vi "OP600ZP_CLUSTER_SOFTS_FIN.vi"(10 "MESURES":T1, 11 "EmptyTab":string[][](array[string])) -> (4 "Tab1":string[][](array[string]), 6 "PASS/FAIL":bool[](array[boolean]))   [LabVIEW 2020]
uses:
  VG/IS30%.vi
  OP600ZP_VGConf.vi
panel:
  out "VG IS30% ?":bool
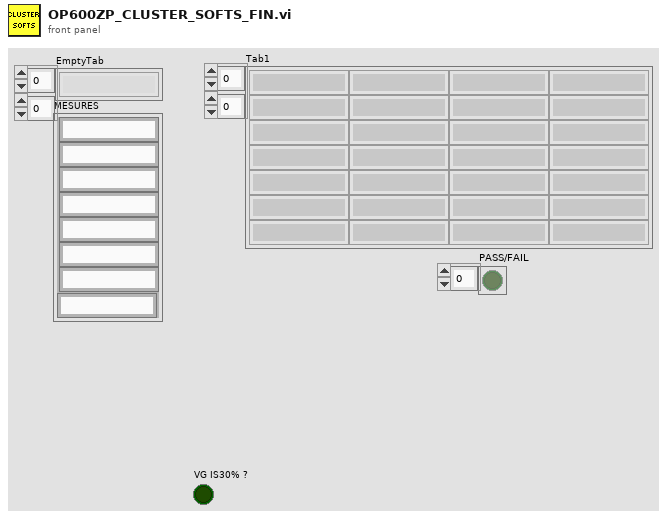
[diagram p1: front panel]
types:
  T1 = cluster{string, string, string, string, string, string, string, string}
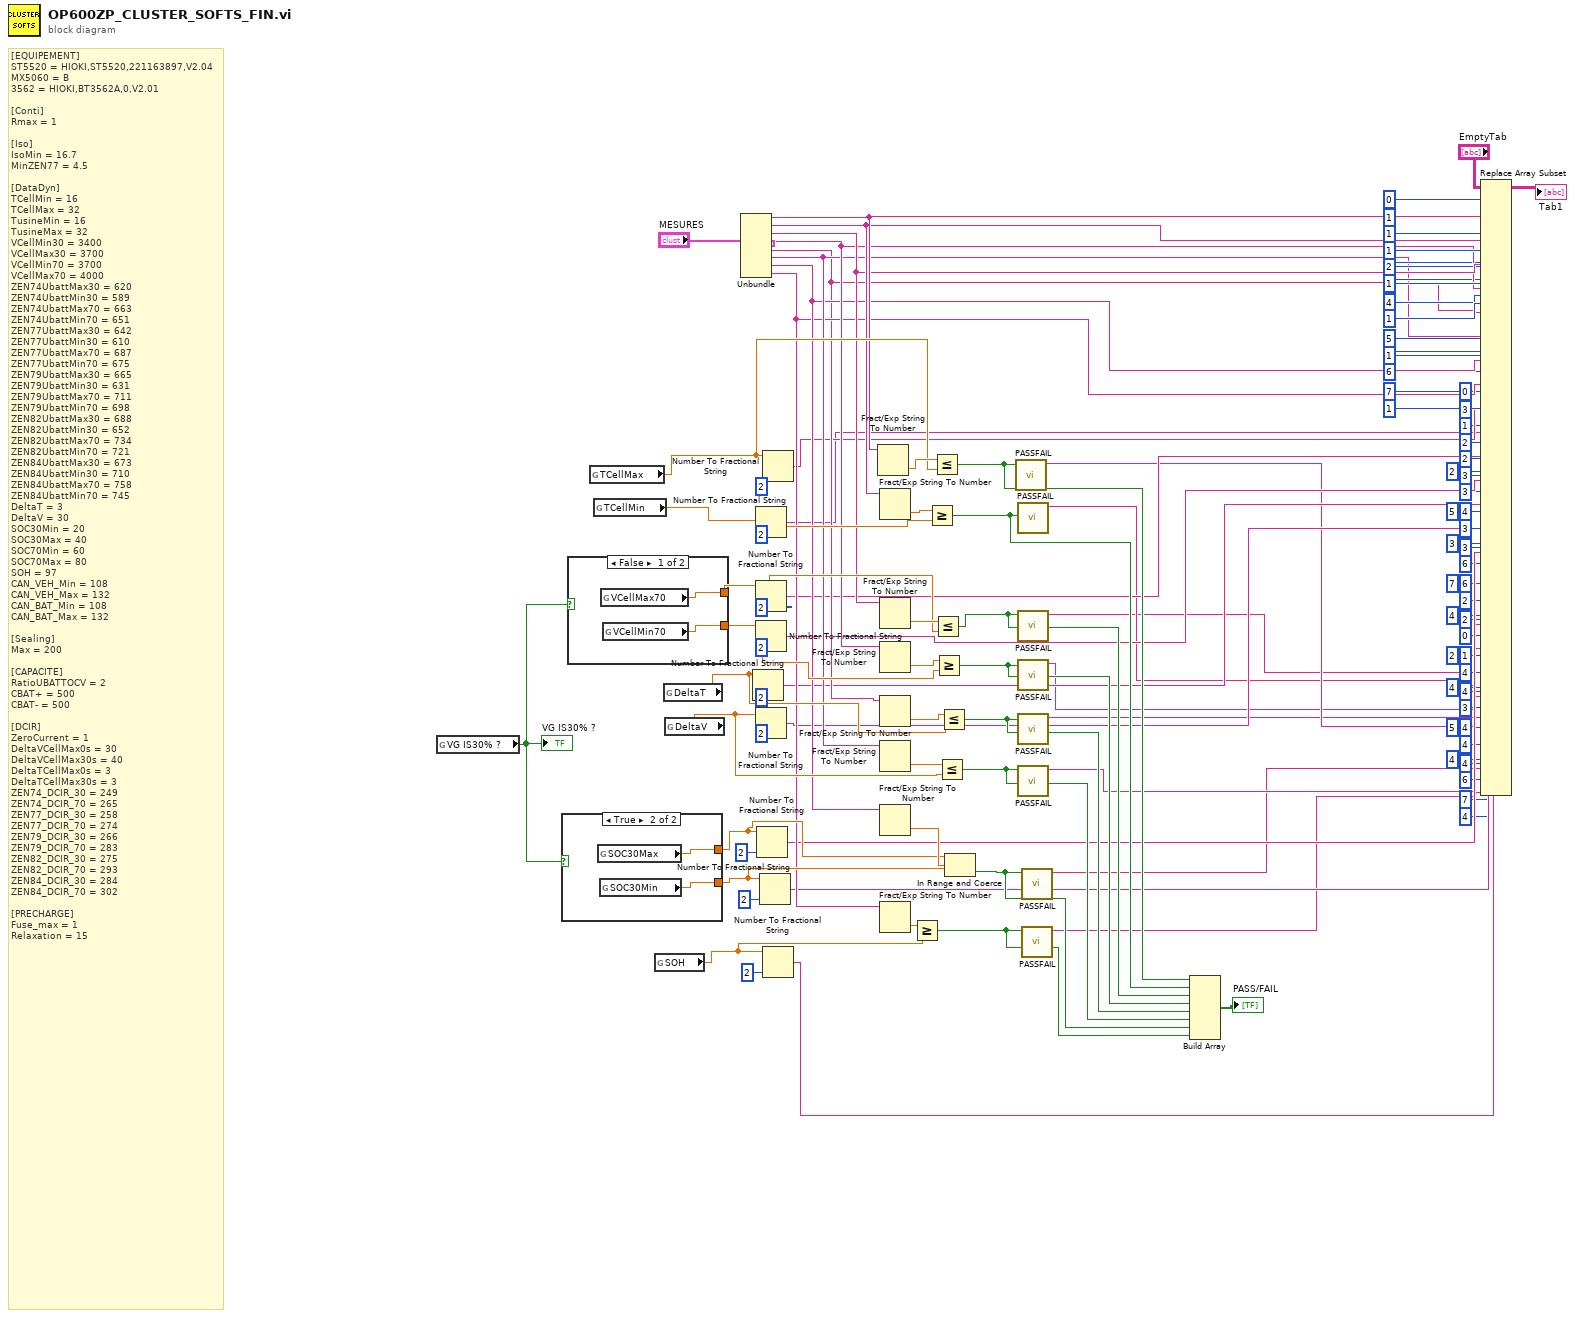
[diagram p0: block diagram]
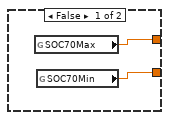
[diagram p2: hidden frame]
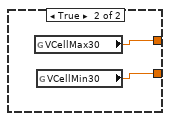
[diagram p3: hidden frame]
diagram:
  # "[EQUIPEMENT]\nST5520 = HIOKI,ST5520,221163897,V2.04\t\nMX5060 = B\n3562 = HIOKI,BT3562A,0,V2.01\n\n[Conti]\nRmax = 1\n\n[Iso]\nIsoMin = 16.7\nMinZEN77 = 4.5\n\n[DataDyn]\nTCellMin = 16\nTCellMax = 32\nTusineMin = 16\nTusineMax = 32\nVCellMin30 = 3400\nVCellMax30 = 3700\nVCellMin70 = 3700\nVCellMax70 = 4000\nZEN74UbattMax30 = 620\nZEN74UbattMin30 = 589\nZEN74UbattMax70 = 663\nZEN74UbattMin70 = 651\nZEN77UbattMax30 = 642\nZEN77UbattMin30 = 610\nZEN77UbattMax70 = 687\nZEN77UbattMin70 = 675\nZEN79UbattMax30 = 665\nZEN79UbattMin30 = 631\nZEN79UbattMax70 = 711\nZEN79UbattMin70 = 698\nZEN82UbattMax30 = 688\nZEN82UbattMin30 = 652\nZEN82UbattMax70 = 734\nZEN82UbattMin70 = 721\nZEN84UbattMax30 = 673\nZEN84UbattMin30 = 710\nZEN84UbattMax70 = 758\nZEN84UbattMin70 = 745\nDeltaT = 3\nDeltaV = 30\nSOC30Min = 20\nSOC30Max = 40\nSOC70Min = 60\nSOC70Max = 80\nSOH = 97\nCAN_VEH_Min = 108\nCAN_VEH_Max = 132\nCAN_BAT_Min = 108\nCAN_BAT_Max = 132\n\n[Sealing]\nMax = 200\n\n[CAPACITE]\nRatioUBATTOCV = 2\nCBAT+ = 500\nCBAT- = 500\n\n[DCIR]\nZeroCurrent = 1\nDeltaVCellMax0s = 30\nDeltaVCellMax30s = 40\nDeltaTCellMax0s = 3\nDeltaTCellMax30s = 3\nZEN74_DCIR_30 = 249\nZEN74_DCIR_70 = 265\nZEN77_DCIR_30 = 258\nZEN77_DCIR_70 = 274\nZEN79_DCIR_30 = 266\nZEN79_DCIR_70 = 283\nZEN82_DCIR_30 = 275\nZEN82_DCIR_70 = 293\nZEN84_DCIR_30 = 284\nZEN84_DCIR_70 = 302\n\n[PRECHARGE]\nFuse_max = 1\nRelaxation = 15"
  n1 = global read "IS30%.vi" "VG IS30% ?"() -> (w94:bool)
  "VG IS30% ?" <- w94
  n2 = case shown="True" w94 {
    tunnel: [w116 w118] -> w87
    tunnel: [w115 w117] -> w86
    frame False {
      n3 = global read "OP600ZP_VGConf.vi" "SOC70Max"() -> (w116:dbl)
      n4 = global read "OP600ZP_VGConf.vi" "SOC70Min"() -> (w115:dbl)
    }
    frame True {
      n5 = global read "OP600ZP_VGConf.vi" "SOC30Max"() -> (w118:dbl)
      n6 = global read "OP600ZP_VGConf.vi" "SOC30Min"() -> (w117:dbl)
    }
  }
  n7 = case shown="False" w94 {
    tunnel: [w120 w122] -> w108
    tunnel: [w119 w121] -> w106
    frame False {
      n8 = global read "OP600ZP_VGConf.vi" "VCellMax70"() -> (w120:dbl)
      n9 = global read "OP600ZP_VGConf.vi" "VCellMin70"() -> (w119:dbl)
    }
    frame True {
      n10 = global read "OP600ZP_VGConf.vi" "VCellMax30"() -> (w122:dbl)
      n11 = global read "OP600ZP_VGConf.vi" "VCellMin30"() -> (w121:dbl)
    }
  }
  n12 = global read "OP600ZP_VGConf.vi" "TCellMax"() -> (w98:dbl)
  n13 = global read "OP600ZP_VGConf.vi" "TCellMin"() -> (w97:dbl)
  n14 = global read "OP600ZP_VGConf.vi" "SOH"() -> (w90:dbl)
  n15 = global read "OP600ZP_VGConf.vi" "DeltaT"() -> (w96:dbl)
  n16 = global read "OP600ZP_VGConf.vi" "DeltaV"() -> (w95:dbl)
  n17 = Unbundle("MESURES") -> (w75:string, w72:string, w69:string, w66:string, w52:string, w61:string, w58:string, w55:string)
  n18 = Number To Fractional String(number=w96, precision (6)=i16 2 ("précision (6)")) -> (F-format string=w39:string)  [unwired: 2 in]
  n19 = Number To Fractional String(number=w97, precision (6)=i16 2 ("précision (6)")) -> (F-format string=w48:string)  [unwired: 2 in]
  n20 = Number To Fractional String(number=w108, precision (6)=i16 2 ("précision (6)")) -> (F-format string=w45:string)  [unwired: 2 in]
  n21 = Number To Fractional String(number=w106, precision (6)=i16 2 ("précision (6)")) -> (F-format string=w42:string)  [unwired: 2 in]
  n22 = Number To Fractional String(number=w95, precision (6)=i16 2 ("précision (6)")) -> (F-format string=w36:string)  [unwired: 2 in]
  n23 = Number To Fractional String(number=w87, precision (6)=i16 2 ("précision (6)")) -> (F-format string=w33:string)  [unwired: 2 in]
  n24 = Number To Fractional String(number=w86, precision (6)=i16 2 ("précision (6)")) -> (F-format string=w30:string)  [unwired: 2 in]
  n25 = Number To Fractional String(number=w98, precision (6)=i16 2 ("précision (6)")) -> (F-format string=w51:string)  [unwired: 2 in]
  n26 = Number To Fractional String(number=w90, precision (6)=i16 2 ("précision (6)")) -> (F-format string=w27:string)  [unwired: 2 in]
  n27 = Fract/Exp String To Number(string=w75) -> (number=w104:dbl)  [unwired: 3 in, 1 out]
  n28 = Fract/Exp String To Number(string=w72) -> (number=w103:dbl)  [unwired: 3 in, 1 out]
  n29 = Fract/Exp String To Number(string=w69) -> (number=w109:dbl)  [unwired: 3 in, 1 out]
  n30 = Fract/Exp String To Number(string=w66) -> (number=w107:dbl)  [unwired: 3 in, 1 out]
  n31 = Fract/Exp String To Number(string=w52) -> (number=w100:dbl)  [unwired: 3 in, 1 out]
  n32 = Fract/Exp String To Number(string=w61) -> (number=w105:dbl)  [unwired: 3 in, 1 out]
  n33 = Fract/Exp String To Number(string=w58) -> (number=w88:dbl)  [unwired: 3 in, 1 out]
  n34 = Fract/Exp String To Number(string=w55) -> (number=w89:dbl)  [unwired: 3 in, 1 out]
  n35 = Greater Or Equal?(x=w89, y=w90) -> (x >= y?=w76:bool)
  n36 = Greater Or Equal?(x=w103, y=w97) -> (x >= y?=w82:bool)
  n37 = Less Or Equal?(x=w104, y=w98) -> (x <= y?=w83:bool)
  n38 = Less Or Equal?(x=w109, y=w108) -> (x <= y?=w81:bool)
  n39 = Greater Or Equal?(x=w107, y=w106) -> (x >= y?=w80:bool)
  n40 = Less Or Equal?(x=w105, y=w95) -> (x <= y?=w78:bool)
  n41 = Less Or Equal?(x=w100, y=w96) -> (x <= y?=w79:bool)
  n42 = In Range and Coerce(upper limit=w87, x=w88, lower limit=w86) -> (In Range?=w77:bool)  [unwired: 1 out]
  n43 = call <userlib>:"PASSFAIL.vi"("E"=w83) -> ("S"=w24:string)  [unwired: 10 in]
  n44 = call <userlib>:"PASSFAIL.vi"("E"=w82) -> ("S"=w21:string)  [unwired: 10 in]
  n45 = call <userlib>:"PASSFAIL.vi"("E"=w81) -> ("S"=w18:string)  [unwired: 10 in]
  n46 = call <userlib>:"PASSFAIL.vi"("E"=w80) -> ("S"=w15:string)  [unwired: 10 in]
  n47 = call <userlib>:"PASSFAIL.vi"("E"=w79) -> ("S"=w12:string)  [unwired: 10 in]
  n48 = call <userlib>:"PASSFAIL.vi"("E"=w78) -> ("S"=w9:string)  [unwired: 10 in]
  n49 = call <userlib>:"PASSFAIL.vi"("E"=w77) -> ("S"=w6:string)  [unwired: 10 in]
  n50 = call <userlib>:"PASSFAIL.vi"("E"=w76) -> ("S"=w3:string)  [unwired: 10 in]
  n51 = Build Array(w83, w82, w81, w80, w79, w78, w77, w76) -> (→"PASS/FAIL":bool[])
  n52 = Replace Array Subset(array="EmptyTab", new element #1=w75, index (row) #1=0 ("indice (ligne)"), index (col) #1=1 ("indice désactivé (col)"), new element #2=w72, index (row) #2=1 ("indice (ligne)"), index (col) #2=1 ("indice désactivé (col)"), new element #3=w69, index (row) #3=2 ("indice (ligne)"), index (col) #3=1 ("indice désactivé (col)"), new element #4=w66, index (row) #4=3 ("indice (ligne)"), index (col) #4=1 ("indice désactivé (col)"), new element #5=w52, index (row) #5=4 ("indice désactivé (ligne)"), index (col) #5=1 ("indice (col)"), new element #6=w61, index (row) #6=5 ("indice (ligne)"), index (col) #6=1 ("indice désactivé (col)"), new element #7=w58, index (row) #7=6 ("indice (ligne)"), index (col) #7=1 ("indice désactivé (col)"), new element #8=w55, index (row) #8=7 ("indice (ligne)"), index (col) #8=1 ("indice désactivé (col)"), new element #9=w51, index (row) #9=0 ("indice (ligne)"), index (col) #9=3 ("indice désactivé (col)"), new element #10=w48, index (row) #10=1 ("indice (ligne)"), index (col) #10=2 ("indice désactivé (col)"), new element #11=w45, index (row) #11=2 ("indice (ligne)"), index (col) #11=3 ("indice désactivé (col)"), new element #12=w42, index (row) #12=3 ("indice (ligne)"), index (col) #12=2 ("indice désactivé (col)"), new element #13=w39, index (row) #13=4 ("indice (ligne)"), index (col) #13=3 ("indice désactivé (col)"), new element #14=w36, index (row) #14=5 ("indice (ligne)"), index (col) #14=3 ("indice désactivé (col)"), new element #15=w33, index (row) #15=6 ("indice (ligne)"), index (col) #15=3 ("indice désactivé (col)"), new element #16=w30, index (row) #16=6 ("indice (ligne)"), index (col) #16=2 ("indice désactivé (col)"), new element #17=w27, index (row) #17=7 ("indice (ligne)"), index (col) #17=2 ("indice désactivé (col)"), new element #18=w24, index (row) #18=0 ("indice (ligne)"), index (col) #18=4 ("indice désactivé (col)"), new element #19=w21, index (row) #19=1 ("indice (ligne)"), index (col) #19=4 ("indice désactivé (col)"), new element #20=w18, index (row) #20=2 ("indice (ligne)"), index (col) #20=4 ("indice désactivé (col)"), new element #21=w15, index (row) #21=3 ("indice (ligne)"), index (col) #21=4 ("indice désactivé (col)"), new element #22=w12, index (row) #22=4 ("indice (ligne)"), index (col) #22=4 ("indice désactivé (col)"), new element #23=w9, index (row) #23=5 ("indice (ligne)"), index (col) #23=4 ("indice désactivé (col)"), new element #24=w6, index (row) #24=6 ("indice (ligne)"), index (col) #24=4 ("indice désactivé (col)"), new element #25=w3, index (row) #25=7 ("indice (ligne)"), index (col) #25=4 ("indice désactivé (col)")) -> (→"Tab1":string[][])
